vi "sub_waypoints_upload_final.vi"(11 "wpt cfg":T1) -> (1 "wpt length":dbl, 2 "Total wpt":cluster{"X":dbl, "Y":dbl}[](array[cluster]), 3 "Total wpt w stoppt":T2(array[cluster]))   [LabVIEW 2019]
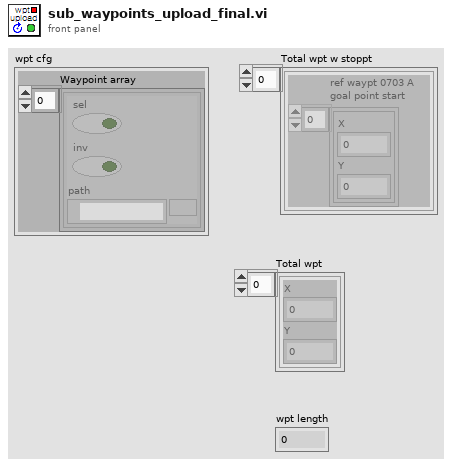
[diagram p1: front panel]
types:
  T1 = cluster{"Waypoint array":cluster{"sel":bool, "inv":bool, "path":path}[]}
  T2 = cluster{"ref waypt 0703 A \ngoal point start":cluster{"X":dbl, "Y":dbl}[]}[]
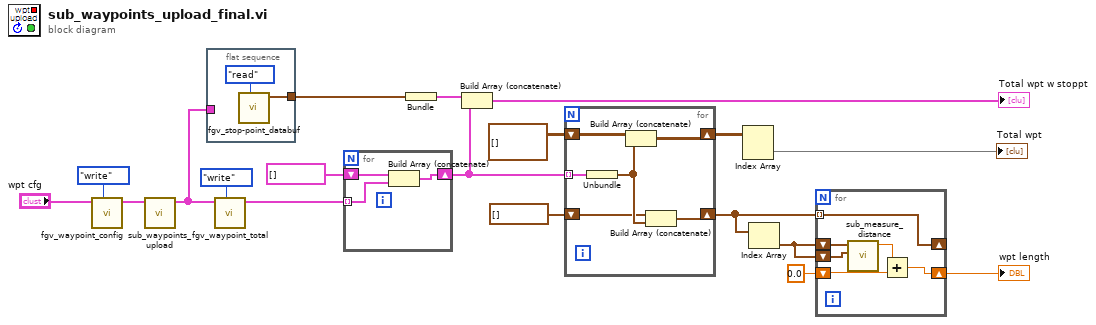
[diagram p0: block diagram]
diagram:
  n1 = call "fgv_waypoint_config.vi"("cmd"=enum16{"read", "write"}."write", "waypoint files cfg"="wpt cfg") -> ("waypoint files cfg out"=w5:T1)  [unwired: 9 in]
  n2 = call "sub_waypoints_upload.vi"("waypoint group"=w5) -> ("waypoint all"=w8:cluster{"XY 그래프":cluster{"X":dbl, "Y":dbl}[]}[])  [unwired: 9 in, 1 out]
  n3 = flat-sequence {
    tunnel: [w20] -> w7
    tunnel: w8 -> [_]
    frame #0 {
      n4 = call "fgv_stop-point_databuf.vi"("cmd"=enum16{"clear", "write", "read"}."read") -> ("all stop pts out"=w20:cluster{dbl, dbl}[])  [unwired: 9 in, 1 out]
    }
  }
  n5 = call "fgv_waypoint_total.vi"("cmd"=enum16{"write", "read"}."write", "waypoint total in"=w8) -> ("waypoint total out"=w9:cluster{"waypt":cluster{"X":dbl, "Y":dbl}[]}[])  [unwired: 9 in]
  n6 = for {
    shift-right: [w22] -> w13
    shift-left: T2 [] -> [w23]
    tunnel: w9 -> [w24] mode=indexing
    n7 = Build Array (concatenate)(w23, w24) -> (w22:cluster{"waypt":cluster{"X":dbl, "Y":dbl}[]}[])
  }
  n8 = Bundle("all stop pts out"=w7) -> (w10:cluster{"all stop pts out":cluster{dbl, dbl}[]})  [unwired: 1 in]
  n9 = Build Array (concatenate)(w10, w13) -> (→"Total wpt w stoppt":T2)
  n10 = for {
    tunnel: w13 -> [w29] mode=indexing
    shift-right: [w30] -> w12
    shift-left: cluster{"X":dbl, "Y":dbl}[][] [] -> [w28]
    shift-right: [w27] -> w16
    shift-left: cluster{"X":dbl, "Y":dbl}[] [] -> [w25]
    n11 = Unbundle(w29) -> ("ref waypt 0703 A \ngoal point start"=w26:cluster{"X":dbl, "Y":dbl}[])
    n12 = Build Array (concatenate)(w28, w26) -> (w30:cluster{"X":dbl, "Y":dbl}[][])
    n13 = Build Array (concatenate)(w25, w26) -> (w27:cluster{"X":dbl, "Y":dbl}[])
  }
  n14 = Index Array(array=w12) -> (element=→"Total wpt":cluster{"X":dbl, "Y":dbl}[])  [unwired: 2 in]
  n15 = Index Array(array=w16) -> (element=w17:cluster{"X":dbl, "Y":dbl})  [unwired: 1 in]
  n16 = for {
    tunnel: w16 -> [w36] mode=indexing
    shift-right: [w36] -> _
    shift-left: w17 -> [w35]
    shift-left: w17 -> [w34]
    shift-right: [w31] -> w19
    shift-left: 0.0 -> [w33]
    n17 = call "sub_measure_distance.vi"("pt 2"=w34, "pt 1"=w35) -> ("distance"=w32:dbl)  [unwired: 9 in]
    n18 = Add(x=w32, y=w33) -> (x+y=w31:dbl)
  }
  "wpt length" <- w19
